vi "Get Return Values.vi"(8 "error in (no error)":errorcluster, 11 "Mock In":refnum<class "Responsive Mock.lvclass">) -> (0 "error out":errorcluster, 2 "Indicator Values":map{string, variant}(c390), 3 "Mock Out":refnum<class "Responsive Mock.lvclass">)   [LabVIEW 2020, in "Responsive Mock.lvclass"]
uses:
  Responsive Mock.lvclass
  Responsive Mock.lvclass/Responsive Mock.ctl
  Core/VI Call/VI Call.lvclass
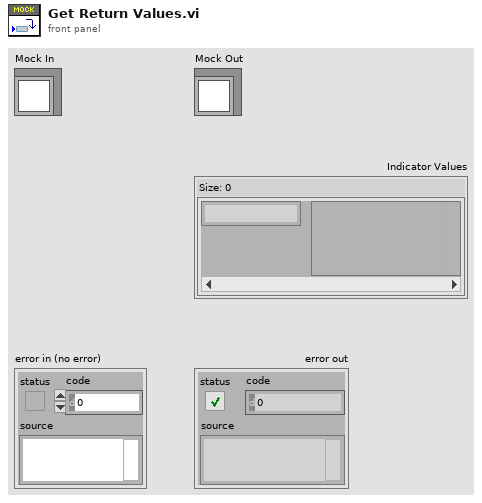
[diagram p1: front panel]
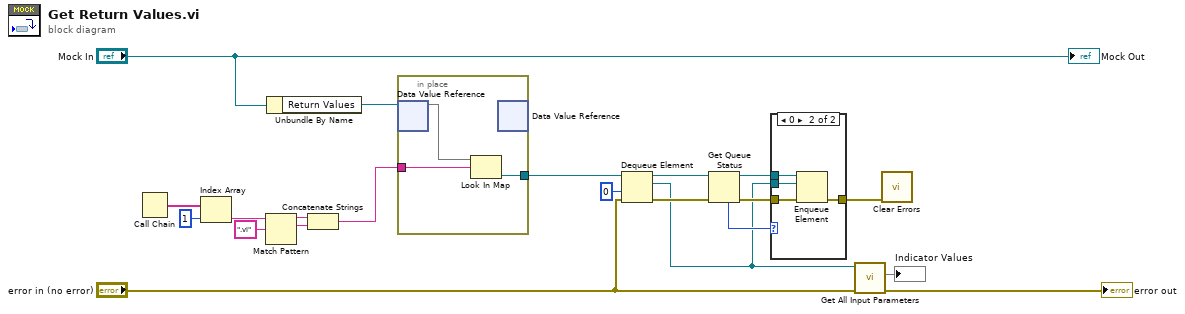
[diagram p0: block diagram]
diagram:
  n1 = Call Chain() -> (call chain=w8:string[])
  n2 = Index Array(array=w8, index=1) -> (element=w3:string)
  n3 = Match Pattern(string=w3, regular expression=".vi") -> (before substring=w5:string, match substring=w4:string)  [unwired: 1 in, 2 out]
  n4 = Unbundle By Name("Mock In") -> ("Return Values"=w19:refnum<data-value>)
  n5 = Concatenate Strings(w5, w4) -> (w2:string)
  n6 = in-place {
    in-place-border: w2 -> [w23]
    in-place-border: [w22] -> w18
    n7 = in-place-dvr #1(w19) -> (w24:map{string, refnum<queue>})  [unwired: 1 out]
    n8 = Look In Map(map=w24, key=w23) -> (value=w22:refnum<queue>)  [unwired: 1 in, 1 out]
    n9 = in-place-dvr #1() -> ()  [unwired: 1 in, 2 out]
  }
  n10 = Dequeue Element(queue=w18, timeout in ms (-1)=0, error in (no error)="error in (no error)") -> (queue out=w14:refnum<queue>, element=w9:refnum<class "VI Call.lvclass">, error out=w16:errorcluster)  [unwired: 1 out]
  n11 = Get Queue Status(queue=w14, error in (no error)=w16) -> (queue out=w12:refnum<queue>, error out=w15:errorcluster, # elements in queue=w11:i32)  [unwired: 1 in, 5 out]
  n12 = case shown="0" w11 {
    tunnel: w15 -> [w25 w29]
    tunnel: [w25 w28] -> w13
    tunnel: w12 -> [_ w27]
    tunnel: w9 -> [_ w26]
    frame Default {
    }
    frame 0 {
      n13 = Enqueue Element(queue=w27, element=w26, error in (no error)=w29) -> (error out=w28:errorcluster)  [unwired: 1 in, 2 out]
    }
  }
  n14 = call-dynamic "Get All Input Parameters.vi"("error in (no error)"="error in (no error)", "VI Call in"=w9) -> ("error out"=→"error out":errorcluster, "Input Parameters"=→"Indicator Values":map{string, variant})  [unwired: 8 in]
  n15 = call <vilib>:"Clear Errors.vi"("error in (no error)"=w13) -> ()  [unwired: 5 in, 2 out]
  "Mock Out" <- "Mock In"
